vi "I2C Line Tracking Example.vi"() -> ()   [LabVIEW 2018]
uses:
  library/Types/Intersection.ctl
  library/Types/Vector.ctl
  <vilib>/Rock Robotics/SystemInterfaces/i2clib/i2c_bus.ctl
  library/Interface/Pixy Com.lvclass
  library/Pixy2.lvlib
  deviceSupport/FRC/I2C/RoboRIO I2C.lvclass
panel:
  in  "Device Address":u8=84 format="%.0x"
  in  "I2C Bus":T1
  out "error out":errorcluster
  out "vectors":T2[](array[typedef])
  out "intersections":T3[](array[typedef])
  in  "feature map":u8=7 format="%.0x"
  in  "features":enum16{"Main Features", "All Features"}(ring)
  out "view":picture
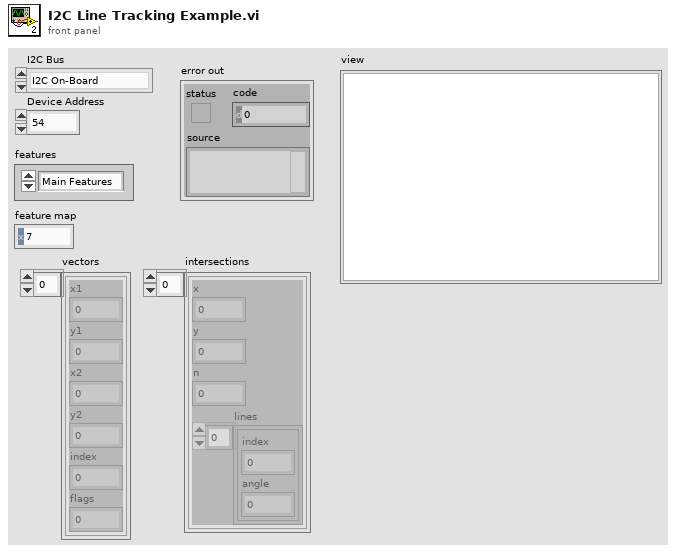
[diagram p1: front panel]
types:
  T1 = typedef "i2c_bus.ctl" = enum16{"I2C On-Board", "I2C MXP", "Invalid"}
  T2 = typedef "Pixy2.lvlib/Vector.ctl" = cluster{"x1":u8, "y1":u8, "x2":u8, "y2":u8, "index":u8, "flags":u8}
  T3 = typedef "Pixy2.lvlib/Intersection.ctl" = cluster{"x":u8, "y":u8, "n":u8, "lines":cluster{"index":u8, "angle":i16}[]}
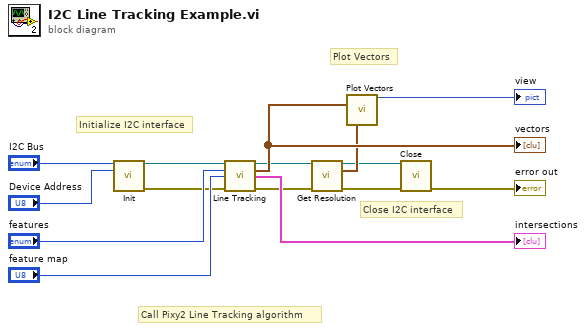
[diagram p0: block diagram]
diagram:
  # "Call Pixy2 Line Tracking algorithm"
  # "Close I2C interface"
  # "Plot Vectors"
  # "Initialize I2C interface"
  n1 = call "Init.vi"("I2C Bus"="I2C Bus", "Device Address"="Device Address") -> ("comm interface out"=w5:refnum<class "Pixy Com.lvclass">, "error out"=w4:errorcluster)  [unwired: 12 in]
  n2 = call "Line Tracking.vi"("comm interface in"=w5, "features"="features", "feature map"="feature map", "error in"=w4) -> ("comm interface out"=w8:refnum<class "Pixy Com.lvclass">, "vectors"=w10:T2[], "intersections"=→"intersections":T3[], "error out"=w7:errorcluster)  [unwired: 7 in, 1 out]
  "vectors" <- w10
  n3 = call "Get Resolution.vi"("comm interface in"=w8, "error in"=w7) -> ("comm interface out"=w2:refnum<class "Pixy Com.lvclass">, "resolution"=w6:cluster{"width":u16, "height":u16}, "error out"=w1:errorcluster)  [unwired: 11 in]
  n4 = call "Plot Vectors.vi"("vectors"=w10, "pixy resolution"=w6) -> ("picture out"=→"view":picture)  [unwired: 13 in]
  n5 = call-dynamic "Close.vi"("comm interface in"=w2, "error in"=w1) -> ("error out"=→"error out":errorcluster)  [unwired: 13 in]
